vi "Setup.vi"(8 "error in (no error)":errorcluster, 11 "LUnit Error Handler Tests In":refnum<class "Error Handler Tests.lvclass">) -> (0 "error out":errorcluster, 3 "LUnit Error Handler Tests Out":refnum<class "Error Handler Tests.lvclass">)   [LabVIEW 2020, in "Error Handler Tests.lvclass"]
doc: "Setup method called by the testing framework before each test method is called."
uses:
  Error Handler Tests.lvclass
  <vilib>/Utility/sysdir.llb/System Directory Type.ctl
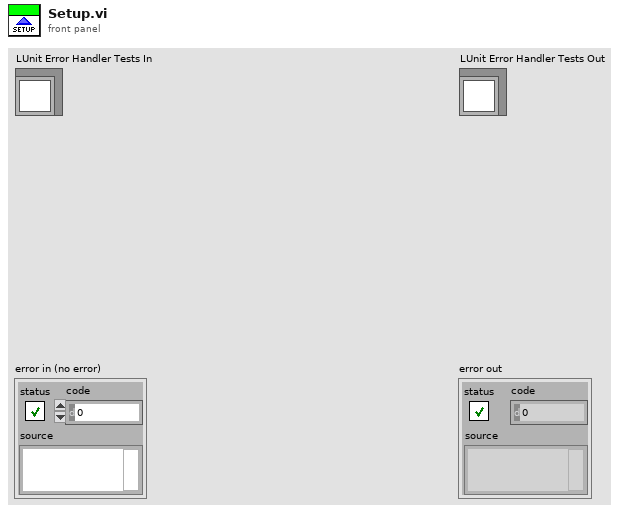
[diagram p1: front panel]
types:
  T1 = typedef "System Directory Type.ctl" = i32
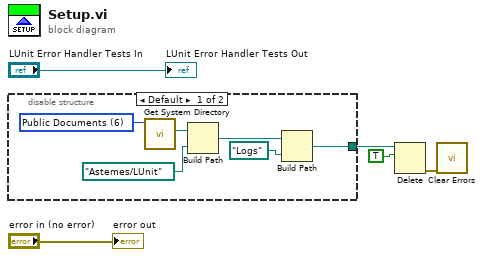
[diagram p0: block diagram]
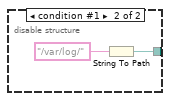
[diagram p2: hidden frame]
diagram:
  n1 = disable-structure shown="Default" {
    disable-tunnel: [w11 w12] -> w2
    frame condition #0 (active) {
      w6 = T1 6 items=["User Home"=0, "User Desktop"=1, "User Documents"=2, "User Application Data"=3, "User Preferences"=4, "User Temporary"=5, "Public Documents"=6, "Public Application Data"=7, "Public Preferences"=8, "Public Cache"=13, "System Core Libraries"=9, "System Installed Libraries"=10, "Application Files"=11, "Boot Volume Root"=12] ("system directory type")
      n2 = call <vilib>:"Get System Directory.vi"("system directory type"=w6) -> ("system directory"=w8:path)  [unwired: 10 in]
      n3 = Build Path(base path=w8, name or relative path=path "Astemes/LUnit") -> (appended path=w9:path)
      n4 = Build Path(base path=w9, name or relative path=path "Logs") -> (appended path=w11:path)
    }
    frame condition #1 {
      n5 = String To Path(string="/var/log/") -> (path=w12:path)
    }
  }
  n6 = Delete(path (use dialog)=w2, entire hierarchy (F)=TRUE) -> (error out=w3:errorcluster)  [unwired: 3 in, 2 out]
  n7 = call <vilib>:"Clear Errors.vi"("error in (no error)"=w3) -> ()  [unwired: 5 in, 2 out]
  "error out" <- "error in (no error)"
  "LUnit Error Handler Tests Out" <- "LUnit Error Handler Tests In"
